vi "AddDefaultBDModules.vi"(6 "error in":errorcluster, 9 "PythonConverter in":refnum<class "PythonBDConverter.lvclass">) -> (0 "error out":errorcluster, 3 "PythonConverter out":refnum<class "PythonBDConverter.lvclass">)   [LabVIEW 2014, in "PythonBDConverter.lvclass"]
uses:
  PythonBDConverter.lvclass
  PythonBDConverter.lvclass/PythonBDConverter.ctl
panel:
  in  "BD modules":T1(array[cluster])=[{"Python module"="pyVI.BD.lvNodes", "Python module  name"="lvNode"}, {"Python module"="pyVI.VI.lvDataTypes", "Python module  name"="lvDT"}, {"Python module"="pyVI.BD.lvStructures", "Python module  name"="lvStruct"}]
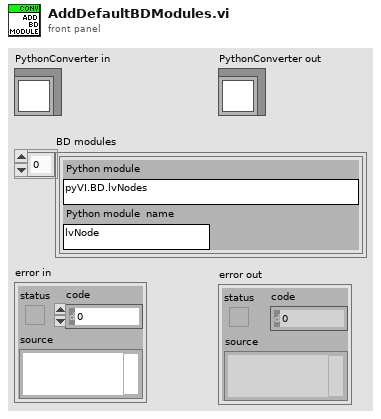
[diagram p1: front panel]
types:
  T1 = cluster{"Python module":string, "Python module  name":string}[]
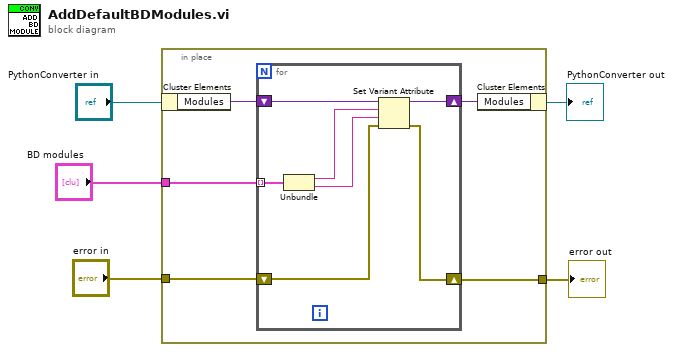
[diagram p0: block diagram]
diagram:
  n1 = in-place {
    in-place-border: "error in" -> [w8]
    in-place-border: [w7] -> w2
    in-place-border: "BD modules" -> [w6]
    n2 = in-place-cluster #1("PythonConverter in") -> ("Modules"=w10:variant)
    n3 = for {
      shift-right: [w16] -> w9
      shift-left: w10 -> [w17]
      shift-right: [w14] -> w7
      shift-left: w8 -> [w15]
      tunnel: w6 -> [w13] mode=indexing
      n4 = Unbundle(w13) -> ("Python module"=w12:string, "Python module  name"=w11:string)
      n5 = Set Variant Attribute(Variant=w17, name=w12, value=w11, error in=w15) -> (Variant out=w16:variant, error out=w14:errorcluster)  [unwired: 1 out]
    }
    n6 = in-place-cluster #1("Modules"=w9) -> (→"PythonConverter out":refnum<class "PythonBDConverter.lvclass">)
  }
  "error out" <- w2
